vi "(SubVI) Decompose filename string to DBL laserpower.vi"(4 "match substring":string="-Stuckbead Scan-", 5 "path":path) -> (1 "LaserPower (mW)":dbl)   [LabVIEW 2014]
panel:
  out "before substring 2":string
  out "match substring":string
  out "before substring":string
  out "after substring":string
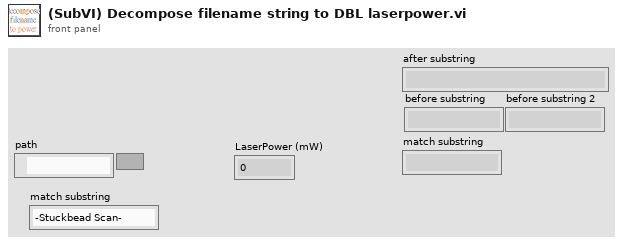
[diagram p1: front panel]
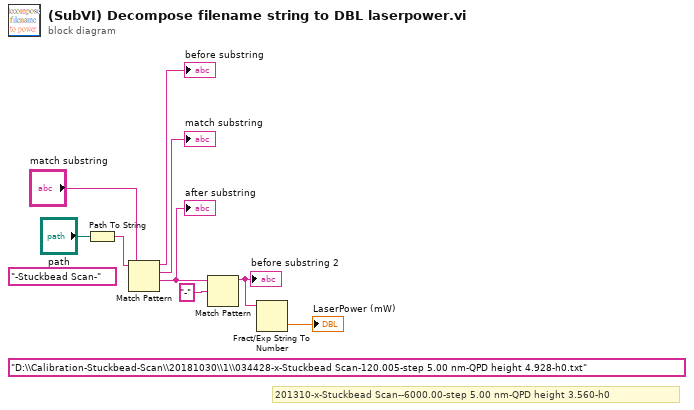
[diagram p0: block diagram]
diagram:
  (unwired) "-Stuckbead Scan-"
  (unwired) "D:\\Calibration-Stuckbead-Scan\\20181030\\1\\034428-x-Stuckbead Scan-120.005-step 5.00 nm-QPD height 4.928-h0.txt"
  # "201310-x-Stuckbead Scan--6000.00-step 5.00 nm-QPD height 3.560-h0"
  n1 = Path To String(path="path") -> (string=w2:string)
  n2 = Match Pattern(string=w2, regular expression="match substring") -> (before substring=→"before substring":string, match substring=→"match substring":string, after substring=w6:string)  [unwired: 1 in, 1 out]
  "after substring" <- w6
  n3 = Match Pattern(string=w6, regular expression="-") -> (before substring=w4:string)  [unwired: 1 in, 3 out]
  "before substring 2" <- w4
  n4 = Fract/Exp String To Number(string=w4) -> (number=→"LaserPower (mW)":dbl)  [unwired: 3 in, 1 out]
